vi "integrationTest.vi"(8 "error in (no error)":errorcluster) -> (0 "error out":errorcluster)   [LabVIEW 2018]
doc: "Execute several tests in TCP client and TCP server."
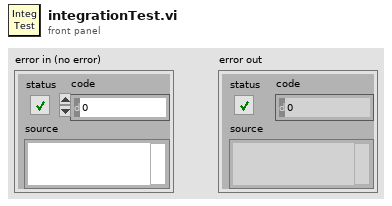
[diagram p1: front panel]
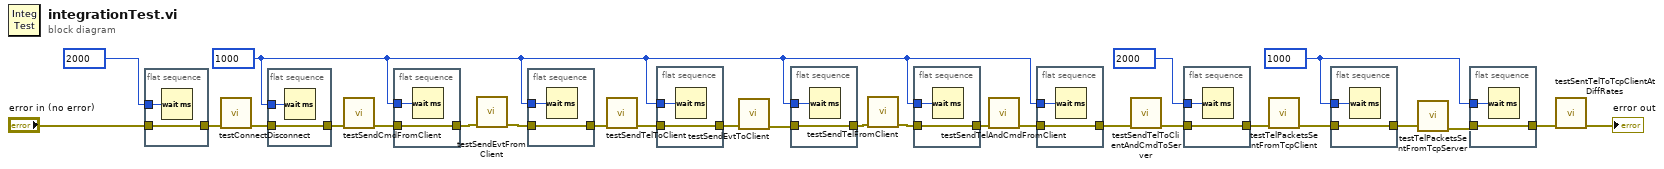
[diagram p0: block diagram]
diagram:
  w4 = u32 1000 ("milliseconds to wait")
  w9 = u32 1000 ("milliseconds to wait")
  n1 = flat-sequence {
    tunnel: [w29] -> w11
    tunnel: "error in (no error)" -> [w29]
    tunnel: u32 2000 ("milliseconds to wait") -> [w28]
    frame #0 {
      n2 = Wait (ms)(milliseconds to wait=w28) -> ()  [unwired: 1 out]
    }
  }
  n3 = call "testConnectDisconnect.vi"("error in (no error)"=w11) -> ("error out"=w27:errorcluster)  [unwired: 10 in]
  n4 = flat-sequence {
    tunnel: [w31] -> w26
    tunnel: w27 -> [w31]
    tunnel: w9 -> [w30]
    frame #0 {
      n5 = Wait (ms)(milliseconds to wait=w30) -> ()  [unwired: 1 out]
    }
  }
  n6 = call "testSendCmdFromClient.vi"("error in (no error)"=w26) -> ("error out"=w25:errorcluster)  [unwired: 10 in]
  n7 = flat-sequence {
    tunnel: [w33] -> w24
    tunnel: w25 -> [w33]
    tunnel: w9 -> [w32]
    frame #0 {
      n8 = Wait (ms)(milliseconds to wait=w32) -> ()  [unwired: 1 out]
    }
  }
  n9 = call "testSendEvtFromClient.vi"("error in (no error)"=w24) -> ("error out"=w23:errorcluster)  [unwired: 10 in]
  n10 = flat-sequence {
    tunnel: [w35] -> w22
    tunnel: w23 -> [w35]
    tunnel: w9 -> [w34]
    frame #0 {
      n11 = Wait (ms)(milliseconds to wait=w34) -> ()  [unwired: 1 out]
    }
  }
  n12 = call "testSendTelToClient.vi"("error in (no error)"=w22) -> ("error out"=w21:errorcluster)  [unwired: 10 in]
  n13 = flat-sequence {
    tunnel: [w37] -> w20
    tunnel: w21 -> [w37]
    tunnel: w9 -> [w36]
    frame #0 {
      n14 = Wait (ms)(milliseconds to wait=w36) -> ()  [unwired: 1 out]
    }
  }
  n15 = call "testSendEvtToClient.vi"("error in (no error)"=w20) -> ("error out"=w19:errorcluster)  [unwired: 10 in]
  n16 = flat-sequence {
    tunnel: [w39] -> w18
    tunnel: w19 -> [w39]
    tunnel: w9 -> [w38]
    frame #0 {
      n17 = Wait (ms)(milliseconds to wait=w38) -> ()  [unwired: 1 out]
    }
  }
  n18 = call "testSendTelFromClient.vi"("error in (no error)"=w18) -> ("error out"=w17:errorcluster)  [unwired: 10 in]
  n19 = flat-sequence {
    tunnel: [w41] -> w16
    tunnel: w17 -> [w41]
    tunnel: w9 -> [w40]
    frame #0 {
      n20 = Wait (ms)(milliseconds to wait=w40) -> ()  [unwired: 1 out]
    }
  }
  n21 = call "testSendTelAndCmdFromClient.vi"("error in (no error)"=w16) -> ("error out"=w15:errorcluster)  [unwired: 10 in]
  n22 = flat-sequence {
    tunnel: [w43] -> w14
    tunnel: w15 -> [w43]
    tunnel: w9 -> [w42]
    frame #0 {
      n23 = Wait (ms)(milliseconds to wait=w42) -> ()  [unwired: 1 out]
    }
  }
  n24 = call "testSendTelToClientAndCmdToServer.vi"("error in (no error)"=w14) -> ("error out"=w13:errorcluster)  [unwired: 10 in]
  n25 = flat-sequence {
    tunnel: w13 -> [w44]
    tunnel: u32 2000 ("milliseconds to wait") -> [w45]
    tunnel: [w44] -> w7
    frame #0 {
      n26 = Wait (ms)(milliseconds to wait=w45) -> ()  [unwired: 1 out]
    }
  }
  n27 = call "testTelPacketsSentFromTcpClient.vi"("error in (no error)"=w7) -> ("error out"=w6:errorcluster)  [unwired: 10 in]
  n28 = flat-sequence {
    tunnel: w6 -> [w46]
    tunnel: w4 -> [w47]
    tunnel: [w46] -> w5
    frame #0 {
      n29 = Wait (ms)(milliseconds to wait=w47) -> ()  [unwired: 1 out]
    }
  }
  n30 = call "testTelPacketsSentFromTcpServer.vi"("error in (no error)"=w5) -> ("error out"=w3:errorcluster)  [unwired: 10 in]
  n31 = flat-sequence {
    tunnel: w3 -> [w48]
    tunnel: w4 -> [w49]
    tunnel: [w48] -> w2
    frame #0 {
      n32 = Wait (ms)(milliseconds to wait=w49) -> ()  [unwired: 1 out]
    }
  }
  n33 = call "testSentTelToTcpClientAtDiffRates.vi"("error in (no error)"=w2) -> ("error out"=→"error out":errorcluster)  [unwired: 10 in]
